vi "SetOutput.vi"(3 "State":bool, 4 "error in":errorcluster, 5 "connection ID":refnum<k5>) -> (1 "error out":errorcluster, 2 "connection ID out":refnum<k5>)   [LabVIEW 2013]
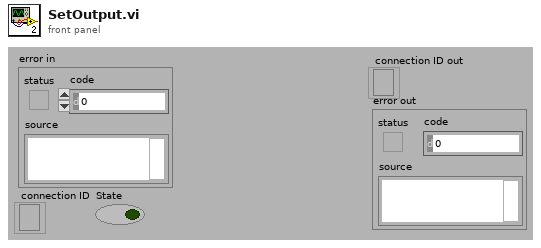
[diagram p1: front panel]
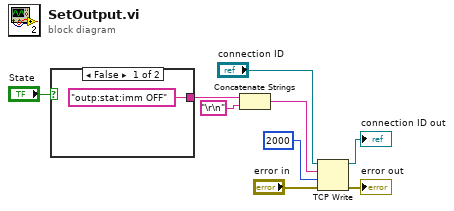
[diagram p0: block diagram]
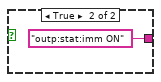
[diagram p2: hidden frame]
diagram:
  n1 = case shown="False" "State" {
    tunnel: ["outp:stat:imm OFF" ("data in") "outp:stat:imm ON" ("data in")] -> w3
    frame False {
    }
    frame True {
    }
  }
  n2 = Concatenate Strings(w3, "\r\n") -> (w2:string)
  n3 = TCP Write(connection ID="connection ID", data in=w2, error in (no error)="error in", 9:2000 ("timeout ms (25000)")) -> (connection ID out=→"connection ID out":refnum<k5>, error out=→"error out":errorcluster)  [unwired: 1 out]
